vi "SpringDamperForceGR.vi"(1 "MotorVelocity":dbl, 2 "MotorPosition":dbl, 4 "SpringDampers":T1(array[cluster])) -> (0 "Force":dbl)   [LabVIEW 2019]
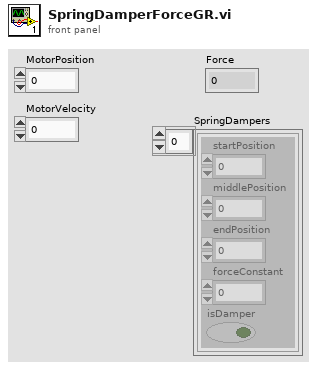
[diagram p1: front panel]
types:
  T1 = cluster{"startPosition":dbl, "middlePosition":dbl, "endPosition":dbl, "forceConstant":dbl, "isDamper":bool}[]
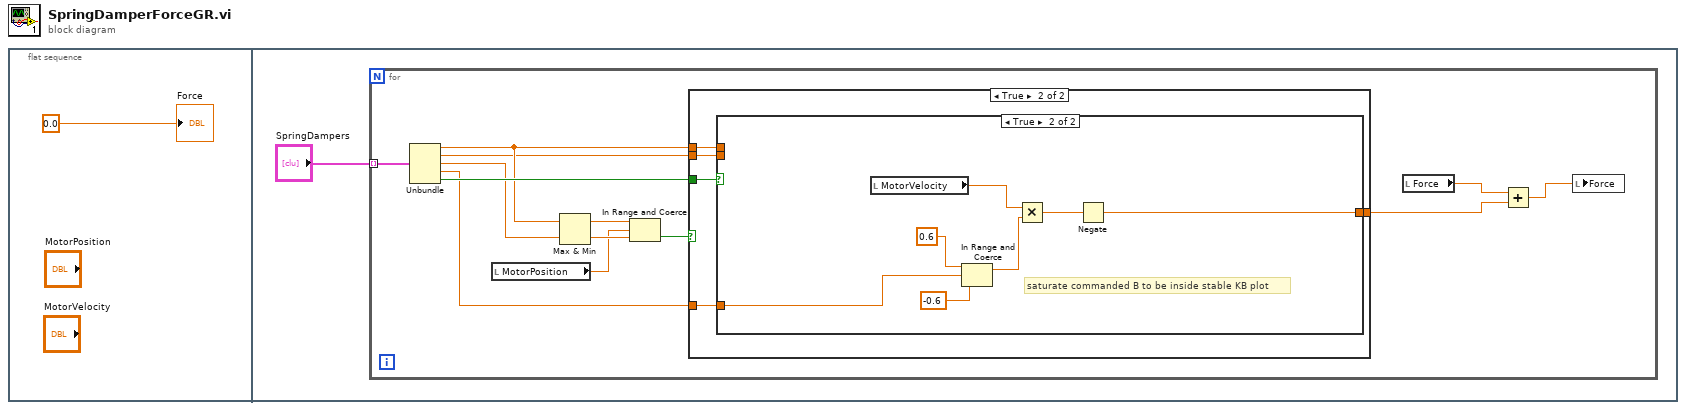
[diagram p0: block diagram]
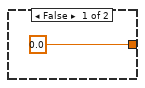
[diagram p2: hidden frame]
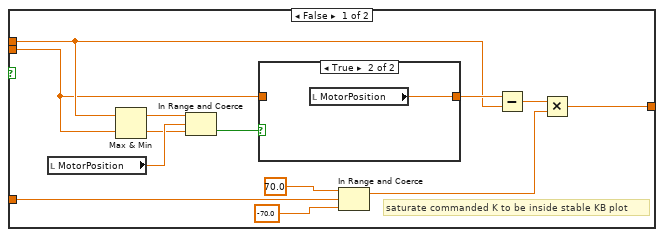
[diagram p3: hidden frame]
diagram:
  n1 = flat-sequence {
    frame #0 {
      "Force" <- 0.0
    }
    frame #1 {
      n2 = for {
        tunnel: "SpringDampers" -> [w15] mode=indexing
        n3 = Unbundle(w15) -> ("startPosition"=w5:dbl, "middlePosition"=w3:dbl, "endPosition"=w4:dbl, "forceConstant"=w6:dbl, "isDamper"=w14:bool)
        n4 = local read "MotorPosition"() -> (w8:dbl)
        n5 = Max & Min(x=w5, y=w4) -> (max(x,y)=w9:dbl, min(x,y)=w10:dbl)
        n6 = In Range and Coerce(upper limit=w9, x=w8, lower limit=w10) -> (In Range?=w11:bool)  [unwired: 1 out]
        n7 = case shown="True" w11 {
          tunnel: w14 -> [_ w21]
          tunnel: [0.0 w19] -> w7
          tunnel: w6 -> [_ w20]
          tunnel: w5 -> [_ w18]
          tunnel: w3 -> [_ w17]
          frame False {
          }
          frame True {
            n8 = case shown="True" w21 {
              tunnel: w20 -> [w25 w37]
              tunnel: [w27 w41] -> w19
              tunnel: w18 -> [w29 _]
              tunnel: w17 -> [w26 _]
              frame False {
                # "saturate commanded K to be inside stable KB plot"
                n9 = local read "MotorPosition"() -> (w34:dbl)
                n10 = Max & Min(x=w29, y=w26) -> (max(x,y)=w33:dbl, min(x,y)=w32:dbl)
                n11 = In Range and Coerce(upper limit=w33, x=w34, lower limit=w32) -> (In Range?=w31:bool)  [unwired: 1 out]
                n12 = case shown="True" w31 {
                  tunnel: [w35 w36] -> w30
                  tunnel: w26 -> [w35 _]
                  frame False {
                  }
                  frame True {
                    n13 = local read "MotorPosition"() -> (w36:dbl)
                  }
                }
                n14 = In Range and Coerce(upper limit=70.0, x=w25, lower limit=-70.0) -> (coerced(x)=w24:dbl)  [unwired: 1 out]
                n15 = Subtract(x=w30, y=w29) -> (x-y=w28:dbl)
                n16 = Multiply(x=w28, y=w24) -> (x*y=w27:dbl)
              }
              frame True {
                # "saturate commanded B to be inside stable KB plot"
                n17 = local read "MotorVelocity"() -> (w43:dbl)
                n18 = In Range and Coerce(upper limit=0.6, x=w37, lower limit=-0.6) -> (coerced(x)=w38:dbl)  [unwired: 1 out]
                n19 = Multiply(x=w43, y=w38) -> (x*y=w42:dbl)
                n20 = Negate(x=w42) -> (-x=w41:dbl)
              }
            }
          }
        }
        n21 = local read "Force"() -> (w13:dbl)
        n22 = Add(x=w13, y=w7) -> (x+y=w12:dbl)
        n23 = local write "Force"(w12) -> ()
      }
    }
  }
